vi "WLM Instantiate.vi"(8 "error in (no error)":errorcluster) -> (0 "error out":errorcluster, 2 "return value":i32)   [LabVIEW 2012]
uses:
  WLM variable typedefs.llb/RFC.ctl
  WLM variable typedefs.llb/Mode.ctl
  WINDOWS/system32/wlmData.dll
panel:
  in  "Mode":T1 items=["cNotifyInstallCallback", "cNotifyRemoveCallback", "cNotifyInstallWaitEvent", "cNotifyRemoveWaitEvent", "cNotifyInstallCallbackEx", "cNotifyInstallWaitEventEx"]
  in  "RFC":T2 items=["cInstCheckForWLM"=-1, "cInstResetCalc"=0, "cInstNotification"=1, "cInstCopyPattern"=2, "cInstControlWLM"=3, "cInstControlDelay"=4, "cInstControlPriority"=5]
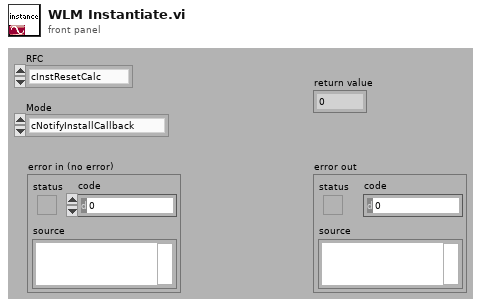
[diagram p1: front panel]
types:
  T1 = typedef "Mode.ctl" = i32
  T2 = typedef "RFC.ctl" = i32
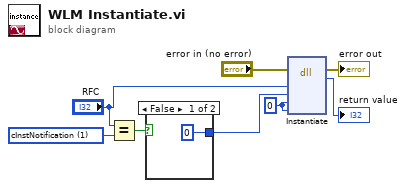
[diagram p0: block diagram]
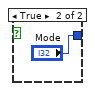
[diagram p2: hidden frame]
diagram:
  w3 = T2 1 items=["cInstCheckForWLM"=-1, "cInstResetCalc"=0, "cInstNotification"=1, "cInstCopyPattern"=2, "cInstControlWLM"=3, "cInstControlDelay"=4, "cInstControlPriority"=5] ("y")
  w7 = 0 ("P2")
  n1 = Equal?(x="RFC", y=w3) -> (x = y?=w4:bool)
  n2 = case shown="False" w4 {
    tunnel: [0 "Mode"] -> w2
    frame False {
    }
    frame True {
    }
  }
  n3 = dll-call lib="C:/WINDOWS/system32/wlmData.dll" fn="Instantiate"(error in="error in (no error)", "RFC"="RFC", "Mode"=w2, "P1"=w7, "P2"=w7) -> (error out=→"error out":errorcluster, "return type"=→"return value":i32)  [unwired: 4 in, 3 out]
